vi "For Loop.vi"() -> ()   [LabVIEW 2015]
panel:
  out "Output 3":dbl
  out "Output 2":dbl
  out "Output":u32
  out "Iterasi":u32
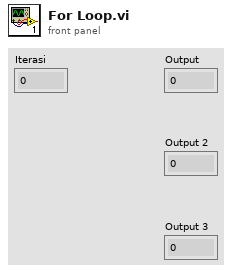
[diagram p1: front panel]
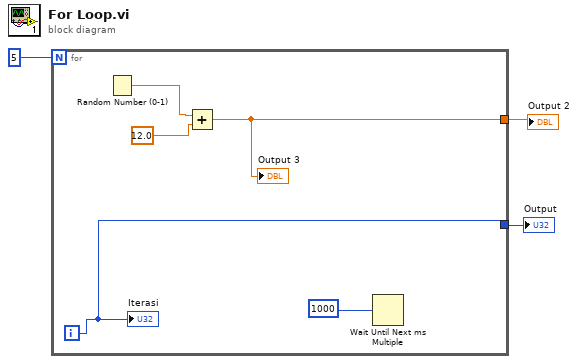
[diagram p0: block diagram]
diagram:
  n1 = for {
    N: 5 -> [_]
    tunnel: [w8] -> w2
    tunnel: [w5] -> w1
    i -> [w8]
    n2 = Random Number (0-1)() -> (number: 0 to 1=w7:dbl)
    n3 = Add(x=w7, y=12.0) -> (x+y=w5:dbl)
    "Output 3" <- w5
    n4 = Wait Until Next ms Multiple(millisecond multiple=1000) -> ()  [unwired: 1 out]
    "Iterasi" <- w8
  }
  "Output" <- w2
  "Output 2" <- w1
